vi "IO_TEST.vi"() -> ()   [LabVIEW 2017]
panel:
  in  "DO_3":bool
  out "status":bool
  in  "SOT READ":bool
  out "SOT":bool
  in  "DO_2":bool
  in  "EOT(DO1)":bool
  in  "stop":bool
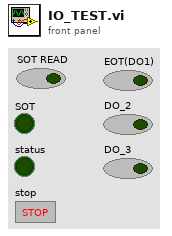
[diagram p1: front panel]
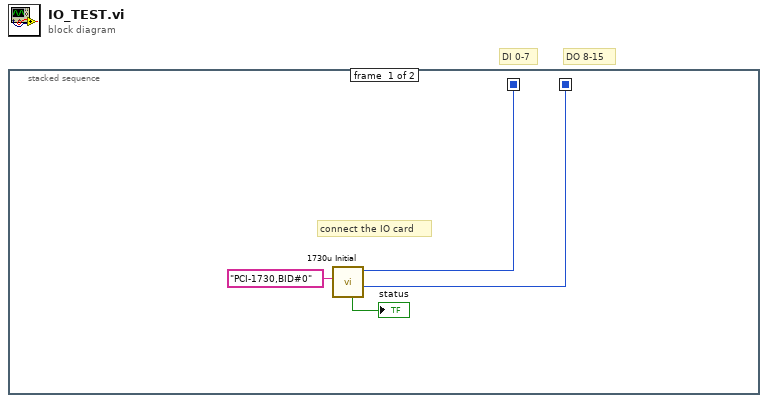
[diagram p0: block diagram]
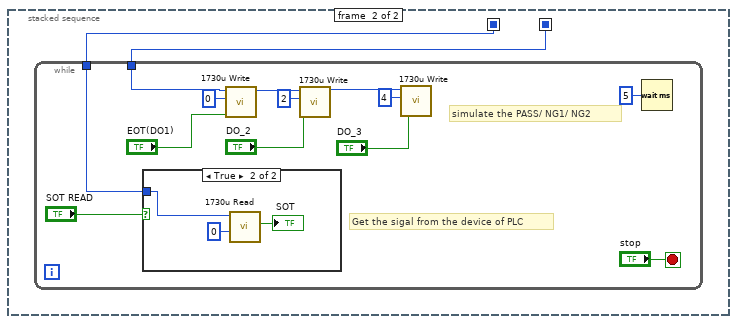
[diagram p2: hidden frame]
diagram:
  # "DO 8-15"
  # "DI 0-7"
  n1 = stacked-sequence {
    seq-local: [w4 _] -> [_ w6]
    seq-local: [w3 _] -> [_ w5]
    frame #0 {
      # "connect the IO card"
      n2 = call <userlib>:"1730u Initial.vi"("physical channels"="PCI-1730,BID#0") -> ("task DO 0~7"=w3:i32, "task DI 0~7"=w4:i32, "status"=→"status":bool)  [unwired: 6 in, 2 out]
    }
    frame #1 {
      n3 = while {
        tunnel: w6 -> [w11]
        tunnel: w5 -> [w14]
        stop <- "stop" stop-if-true
        # "Get the sigal from the device of PLC"
        # "simulate the PASS/ NG1/ NG2"
        n4 = case shown="True" "SOT READ" {
          tunnel: w11 -> [_ w21]
          frame False {
          }
          frame True {
            n5 = call <userlib>:"1730u Read.vi"("portBit"=0, "DI task in"=w21) -> ("data"=→"SOT":bool)  [unwired: 8 in, 1 out]
          }
        }
        n6 = call <userlib>:"1730u Write.vi"("data"="EOT(DO1)", "portBit"=0, "DO task in"=w14) -> ("DO task out"=w16:i32)  [unwired: 8 in]
        n7 = call <userlib>:"1730u Write.vi"("data"="DO_2", "portBit"=2, "DO task in"=w16) -> ("DO task out"=w8:i32)  [unwired: 8 in]
        n8 = call <userlib>:"1730u Write.vi"("data"="DO_3", "portBit"=4, "DO task in"=w8) -> ()  [unwired: 8 in, 1 out]
        n9 = Wait (ms)(milliseconds to wait=u32 5) -> ()  [unwired: 1 out]
      }
    }
  }
